vi "PhidgetResetLibrary.vi"(8 "error in":errorcluster) -> (0 "error out":errorcluster)   [LabVIEW 2012, in "Phidget Common.lvlib"]
doc: "Manually run this VI when any VI using Phidgets has been aborted before all Phidgets could be properly closed. This VI resets the Phidget library to its default state, preventing the need to restart LabVIEW.\n\nNote that resetting the library will close all Phidgets, and it is advised against using this VI while other Phidgets are still running."
uses:
  <instrlib>/Phidgets/Phidget Common/Phidget Common.lvlib
  phidget22.dll
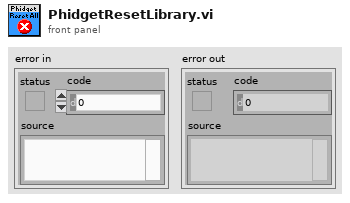
[diagram p1: front panel]
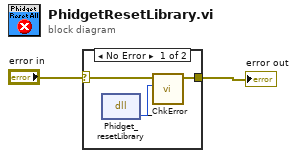
[diagram p0: block diagram]
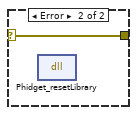
[diagram p2: hidden frame]
diagram:
  n1 = case shown="No Error" "error in" {
    selector: "error in" -> [w5 w6]
    tunnel: [w3 w6] -> w1
    frame No Error {
      n2 = dll-call lib="phidget22.dll" fn="Phidget_resetLibrary"() -> ("return type"=w4:i32)  [unwired: 3 in, 2 out]
      n3 = call <instrlib>:"_ChkError.vi"("Return Code"=w4, "error in (no error)"=w5) -> ("error out"=w3:errorcluster)  [unwired: 9 in]
    }
    frame Error {
      n4 = dll-call lib="phidget22.dll" fn="Phidget_resetLibrary"() -> ()  [unwired: 4 in, 2 out]
    }
  }
  "error out" <- w1
